vi "Read Include or Exclude.vi"(11 "Base Filter in":refnum<class "Base Filter.lvclass">) -> (2 "Include or Exclude":enum16{"Include", "Exclude"}(ring))   [LabVIEW 2016, in "Assert API Components.lvlib" / "Base Filter.lvclass"]
uses:
  Base Filter.lvclass
  Base Filter.lvclass/Base Filter.ctl
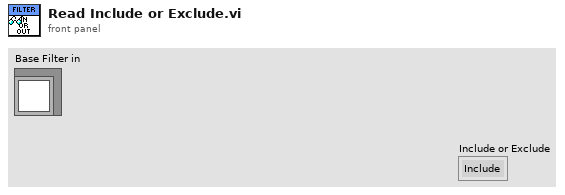
[diagram p1: front panel]
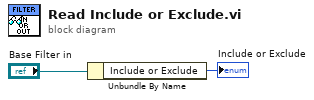
[diagram p0: block diagram]
diagram:
  n1 = Unbundle By Name("Base Filter in") -> ("Include or Exclude"=→"Include or Exclude":enum16{"Include", "Exclude"})
